vi "VI Tree.vi"   [LabVIEW 2010, in "Newport ESP301.lvlib"]
doc: "This is the instrument driver for the <INSTRUMENT NAME>. The VI Tree displays all the user-callable VIs of the instrument driver in an organized table.\n\nNOTE :\nEvery VIs need the VISA Ressource Name parameter for working."
uses:
  <userlib>/Newport ESP301/Newport ESP301.lvlib
panel:
  # "(c) 2009 <Newport>.  ALL RIGHTS RESERVED."
  # "SEE DIAGRAM\nFOR VI TREE."
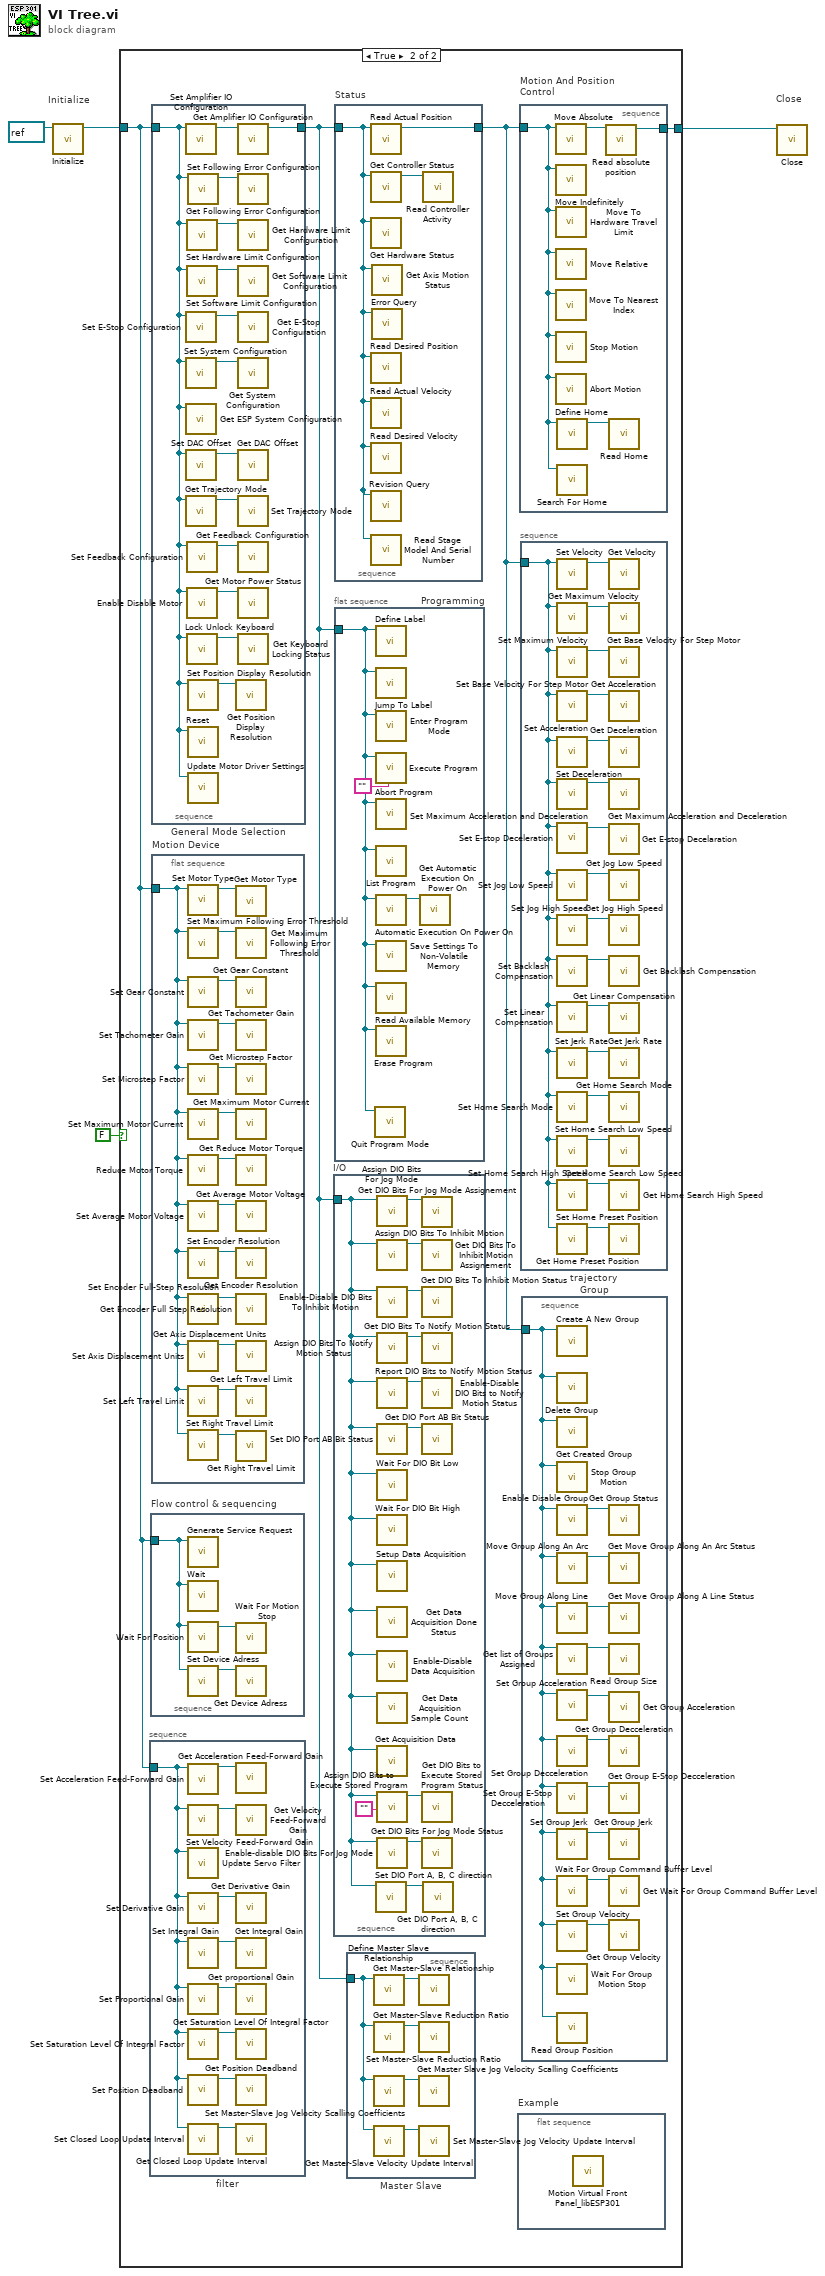
[diagram p0: block diagram]
diagram:
  # "Close"
  # "Initialize"
  n1 = call <userlib>:"Initialize.vi"("VISA resource name"=refnum<visa-resource-name> refnum) -> ("VISA resource name out"=w3:refnum<visa-resource-name>)  [unwired: 8 in, 1 out]
  n2 = case shown="True" FALSE {
    tunnel: w3 -> [w5 w8]
    tunnel: [w5 w6] -> w2
    frame False {
    }
    frame True {
      n3 = stacked-sequence "filter" {
        tunnel: w8 -> [w65]
        frame #0 {
          n4 = call <userlib>:"Set Acceleration Feed-Forward Gain.vi"("VISA resource name"=w65) -> ("VISA resource name out"=w66:refnum<visa-resource-name>)  [unwired: 5 in, 1 out]
          n5 = call <userlib>:"Set Velocity Feed-Forward Gain.vi"("VISA resource name"=w65) -> ("VISA resource name out"=w67:refnum<visa-resource-name>)  [unwired: 5 in, 1 out]
          n6 = call <userlib>:"Update Servo Filter.vi"("VISA resource name"=w65) -> ()  [unwired: 5 in, 2 out]
          n7 = call <userlib>:"Set Derivative Gain.vi"("VISA resource name"=w65) -> ("VISA resource name out"=w71:refnum<visa-resource-name>)  [unwired: 5 in, 1 out]
          n8 = call <userlib>:"Set Integral Gain.vi"("VISA resource name"=w65) -> ("VISA resource name out"=w72:refnum<visa-resource-name>)  [unwired: 5 in, 1 out]
          n9 = call <userlib>:"Set Proportional Gain.vi"("VISA resource name"=w65) -> ("VISA resource name out"=w70:refnum<visa-resource-name>)  [unwired: 5 in, 1 out]
          n10 = call <userlib>:"Set Saturation Level Of Integral Factor.vi"("VISA resource name"=w65) -> ("VISA resource name out"=w69:refnum<visa-resource-name>)  [unwired: 5 in, 1 out]
          n11 = call <userlib>:"Set Position Deadband.vi"("VISA resource name"=w65) -> ("VISA resource name out"=w68:refnum<visa-resource-name>)  [unwired: 5 in, 1 out]
          n12 = call <userlib>:"Set Closed Loop Update Interval.vi"("VISA resource name"=w65) -> ("VISA resource name out"=w64:refnum<visa-resource-name>)  [unwired: 5 in, 1 out]
          n13 = call <userlib>:"Get Acceleration Feed-Forward Gain.vi"("VISA resource name"=w66) -> ()  [unwired: 4 in, 3 out]
          n14 = call <userlib>:"Get Velocity Feed-Forward Gain.vi"("VISA resource name"=w67) -> ()  [unwired: 4 in, 3 out]
          n15 = call <userlib>:"Get Derivative Gain.vi"("VISA resource name"=w71) -> ()  [unwired: 4 in, 3 out]
          n16 = call <userlib>:"Get Integral Gain.vi"("VISA resource name"=w72) -> ()  [unwired: 4 in, 3 out]
          n17 = call <userlib>:"Get proportional Gain.vi"("VISA resource name"=w70) -> ()  [unwired: 4 in, 3 out]
          n18 = call <userlib>:"Get Saturation Level Of Integral Factor.vi"("VISA resource name"=w69) -> ()  [unwired: 4 in, 3 out]
          n19 = call <userlib>:"Get Position Deadband.vi"("VISA resource name"=w68) -> ()  [unwired: 4 in, 3 out]
          n20 = call <userlib>:"Get Closed Loop Update Interval.vi"("VISA resource name"=w64) -> ()  [unwired: 4 in, 3 out]
        }
      }
      n21 = stacked-sequence "Flow control & sequencing" {
        tunnel: w8 -> [w36]
        frame #0 {
          n22 = call <userlib>:"Generate Service Request.vi"("VISA resource name"=w36) -> ()  [unwired: 5 in, 2 out]
          n23 = call <userlib>:"Wait.vi"("VISA resource name"=w36) -> ()  [unwired: 5 in, 2 out]
          n24 = call <userlib>:"Wait For Position.vi"("VISA resource name"=w36) -> ("VISA resource name out"=w38:refnum<visa-resource-name>)  [unwired: 5 in, 1 out]
          n25 = call <userlib>:"Set Device Adress.vi"("VISA resource name"=w36) -> ("VISA resource name out"=w37:refnum<visa-resource-name>)  [unwired: 5 in, 1 out]
          n26 = call <userlib>:"Wait For Motion Stop.vi"("VISA resource name"=w38) -> ()  [unwired: 5 in, 2 out]
          n27 = call <userlib>:"Get Device Adress.vi"("VISA resource name"=w37) -> ()  [unwired: 4 in, 3 out]
        }
      }
      n28 = stacked-sequence "General Mode Selection" {
        tunnel: w8 -> [w23]
        tunnel: [w22] -> w7
        frame #0 {
          n29 = call <userlib>:"Set Amplifier IO Configuration.vi"("VISA resource name"=w23) -> ("VISA resource name out"=w31:refnum<visa-resource-name>)  [unwired: 5 in, 1 out]
          n30 = call <userlib>:"Set E-Stop Configuration.vi"("VISA resource name"=w23) -> ("VISA resource name out"=w32:refnum<visa-resource-name>)  [unwired: 5 in, 1 out]
          n31 = call <userlib>:"Set System Configuration.vi"("VISA resource name"=w23) -> ("VISA resource name out"=w28:refnum<visa-resource-name>)  [unwired: 5 in, 1 out]
          n32 = call <userlib>:"Get ESP System Configuration.vi"("VISA resource name"=w23) -> ()  [unwired: 4 in, 3 out]
          n33 = call <userlib>:"Set DAC Offset.vi"("VISA resource name"=w23) -> ("VISA resource name out"=w30:refnum<visa-resource-name>)  [unwired: 5 in, 1 out]
          n34 = call <userlib>:"Get Trajectory Mode.vi"("VISA resource name"=w23) -> ("VISA resource name out"=w29:refnum<visa-resource-name>)  [unwired: 4 in, 2 out]
          n35 = call <userlib>:"Set Hardware Limit Configuration.vi"("VISA resource name"=w23) -> ("VISA resource name out"=w35:refnum<visa-resource-name>)  [unwired: 5 in, 1 out]
          n36 = call <userlib>:"Set Software Limit Configuration.vi"("VISA resource name"=w23) -> ("VISA resource name out"=w33:refnum<visa-resource-name>)  [unwired: 5 in, 1 out]
          n37 = call <userlib>:"Set Feedback Configuration.vi"("VISA resource name"=w23) -> ("VISA resource name out"=w27:refnum<visa-resource-name>)  [unwired: 5 in, 1 out]
          n38 = call <userlib>:"Enable Disable Motor.vi"("VISA resource name"=w23) -> ("VISA resource name out"=w26:refnum<visa-resource-name>)  [unwired: 5 in, 1 out]
          n39 = call <userlib>:"Lock Unlock Keyboard.vi"("VISA resource name"=w23) -> ("VISA resource name out"=w25:refnum<visa-resource-name>)  [unwired: 5 in, 1 out]
          n40 = call <userlib>:"Set Following Error Configuration.vi"("VISA resource name"=w23) -> ("VISA resource name out"=w34:refnum<visa-resource-name>)  [unwired: 5 in, 1 out]
          n41 = call <userlib>:"Set Position Display Resolution.vi"("VISA resource name"=w23) -> ("VISA resource name out"=w24:refnum<visa-resource-name>)  [unwired: 5 in, 1 out]
          n42 = call <userlib>:"Reset.vi"("VISA resource name"=w23) -> ()  [unwired: 5 in, 2 out]
          n43 = call <userlib>:"Update Motor Driver Settings.vi"("VISA resource name"=w23) -> ()  [unwired: 5 in, 2 out]
          n44 = call <userlib>:"Get Position Display Resolution.vi"("VISA resource name"=w24) -> ()  [unwired: 4 in, 3 out]
          n45 = call <userlib>:"Get Amplifier IO Configuration.vi"("VISA resource name"=w31) -> ("VISA resource name out"=w22:refnum<visa-resource-name>)  [unwired: 4 in, 2 out]
          n46 = call <userlib>:"Get Following Error Configuration.vi"("VISA resource name"=w34) -> ()  [unwired: 4 in, 3 out]
          n47 = call <userlib>:"Get Hardware Limit Configuration.vi"("VISA resource name"=w35) -> ()  [unwired: 4 in, 3 out]
          n48 = call <userlib>:"Get Software Limit Configuration.vi"("VISA resource name"=w33) -> ()  [unwired: 4 in, 3 out]
          n49 = call <userlib>:"Get E-Stop Configuration.vi"("VISA resource name"=w32) -> ()  [unwired: 4 in, 3 out]
          n50 = call <userlib>:"Get System Configuration.vi"("VISA resource name"=w28) -> ()  [unwired: 4 in, 3 out]
          n51 = call <userlib>:"Get DAC Offset.vi"("VISA resource name"=w30) -> ()  [unwired: 4 in, 3 out]
          n52 = call <userlib>:"Set Trajectory Mode.vi"("VISA resource name"=w29) -> ()  [unwired: 6 in, 2 out]
          n53 = call <userlib>:"Get Feedback Configuration.vi"("VISA resource name"=w27) -> ()  [unwired: 4 in, 3 out]
          n54 = call <userlib>:"Get Motor Power Status.vi"("VISA resource name"=w26) -> ()  [unwired: 4 in, 3 out]
          n55 = call <userlib>:"Get Keyboard Locking Status.vi"("VISA resource name"=w25) -> ()  [unwired: 4 in, 3 out]
        }
      }
      n56 = flat-sequence "Motion Device" {
        tunnel: w8 -> [w91]
        frame #0 {
          n57 = call <userlib>:"Set Motor Type.vi"("VISA resource name"=w91) -> ("VISA resource name out"=w103:refnum<visa-resource-name>)  [unwired: 6 in, 1 out]
          n58 = call <userlib>:"Set Maximum Following Error Threshold.vi"("VISA resource name"=w91) -> ("VISA resource name out"=w102:refnum<visa-resource-name>)  [unwired: 5 in, 1 out]
          n59 = call <userlib>:"Set Gear Constant.vi"("VISA resource name"=w91) -> ("VISA resource name out"=w99:refnum<visa-resource-name>)  [unwired: 5 in, 1 out]
          n60 = call <userlib>:"Set Tachometer Gain.vi"("VISA resource name"=w91) -> ("VISA resource name out"=w101:refnum<visa-resource-name>)  [unwired: 5 in, 1 out]
          n61 = call <userlib>:"Set Microstep Factor.vi"("VISA resource name"=w91) -> ("VISA resource name out"=w100:refnum<visa-resource-name>)  [unwired: 5 in, 1 out]
          n62 = call <userlib>:"Set Maximum Motor Current.vi"("VISA resource name"=w91) -> ("VISA resource name out"=w90:refnum<visa-resource-name>)  [unwired: 5 in, 1 out]
          n63 = call <userlib>:"Reduce Motor Torque.vi"("VISA resource name"=w91) -> ("VISA resource name out"=w98:refnum<visa-resource-name>)  [unwired: 6 in, 1 out]
          n64 = call <userlib>:"Set Average Motor Voltage.vi"("VISA resource name"=w91) -> ("VISA resource name out"=w97:refnum<visa-resource-name>)  [unwired: 5 in, 1 out]
          n65 = call <userlib>:"Set Encoder Resolution.vi"("VISA resource name"=w91) -> ("VISA resource name out"=w96:refnum<visa-resource-name>)  [unwired: 5 in, 1 out]
          n66 = call <userlib>:"Set Encoder Full-Step Resolution.vi"("VISA resource name"=w91) -> ("VISA resource name out"=w95:refnum<visa-resource-name>)  [unwired: 5 in, 1 out]
          n67 = call <userlib>:"Set Axis Displacement Units.vi"("VISA resource name"=w91) -> ("VISA resource name out"=w92:refnum<visa-resource-name>)  [unwired: 6 in, 1 out]
          n68 = call <userlib>:"Set Left Travel Limit.vi"("VISA resource name"=w91) -> ("VISA resource name out"=w94:refnum<visa-resource-name>)  [unwired: 5 in, 1 out]
          n69 = call <userlib>:"Set Right Travel Limit.vi"("VISA resource name"=w91) -> ("VISA resource name out"=w93:refnum<visa-resource-name>)  [unwired: 5 in, 1 out]
          n70 = call <userlib>:"Get Motor Type.vi"("VISA resource name"=w103) -> ()  [unwired: 4 in, 3 out]
          n71 = call <userlib>:"Get Maximum Following Error Threshold.vi"("VISA resource name"=w102) -> ()  [unwired: 4 in, 3 out]
          n72 = call <userlib>:"Get Gear Constant.vi"("VISA resource name"=w99) -> ()  [unwired: 4 in, 3 out]
          n73 = call <userlib>:"Get Tachometer Gain.vi"("VISA resource name"=w101) -> ()  [unwired: 4 in, 3 out]
          n74 = call <userlib>:"Get Microstep Factor.vi"("VISA resource name"=w100) -> ()  [unwired: 4 in, 3 out]
          n75 = call <userlib>:"Get Maximum Motor Current.vi"("VISA resource name"=w90) -> ()  [unwired: 4 in, 3 out]
          n76 = call <userlib>:"Get Reduce Motor Torque.vi"("VISA resource name"=w98) -> ()  [unwired: 4 in, 3 out]
          n77 = call <userlib>:"Get Average Motor Voltage.vi"("VISA resource name"=w97) -> ()  [unwired: 4 in, 3 out]
          n78 = call <userlib>:"Get Encoder Resolution.vi"("VISA resource name"=w96) -> ()  [unwired: 4 in, 3 out]
          n79 = call <userlib>:"Get Encoder Full Step Resolution.vi"("VISA resource name"=w95) -> ()  [unwired: 4 in, 3 out]
          n80 = call <userlib>:"Get Axis Displacement Units.vi"("VISA resource name"=w92) -> ()  [unwired: 4 in, 3 out]
          n81 = call <userlib>:"Get Left Travel Limit.vi"("VISA resource name"=w94) -> ()  [unwired: 4 in, 3 out]
          n82 = call <userlib>:"Get Right Travel Limit.vi"("VISA resource name"=w93) -> ()  [unwired: 4 in, 3 out]
        }
      }
      n83 = stacked-sequence "I/O" {
        tunnel: w7 -> [w42]
        frame #0 {
          n84 = call <userlib>:"Set DIO Port A, B, C direction.vi"("VISA resource name"=w42) -> ("VISA resource name out"=w43:refnum<visa-resource-name>)  [unwired: 9 in, 1 out]
          n85 = call <userlib>:"Assign DIO Bits For Jog Mode.vi"("VISA resource name"=w42) -> ("VISA resource name out"=w52:refnum<visa-resource-name>)  [unwired: 6 in, 1 out]
          n86 = call <userlib>:"Assign DIO Bits To Inhibit Motion.vi"("VISA resource name"=w42) -> ("VISA resource name out"=w47:refnum<visa-resource-name>)  [unwired: 6 in, 1 out]
          n87 = call <userlib>:"Enable-Disable DIO Bits To Inhibit Motion.vi"("VISA resource name"=w42) -> ("VISA resource name out"=w48:refnum<visa-resource-name>)  [unwired: 5 in, 1 out]
          n88 = call <userlib>:"Assign DIO Bits To Notify Motion Status.vi"("VISA resource name"=w42) -> ("VISA resource name out"=w49:refnum<visa-resource-name>)  [unwired: 6 in, 1 out]
          n89 = call <userlib>:"Report DIO Bits to Notify Motion Status.vi"("VISA resource name"=w42) -> ("VISA resource name out"=w51:refnum<visa-resource-name>)  [unwired: 4 in, 2 out]
          n90 = call <userlib>:"Set DIO Port AB Bit Status.vi"("VISA resource name"=w42) -> ("VISA resource name out"=w50:refnum<visa-resource-name>)  [unwired: 5 in, 1 out]
          n91 = call <userlib>:"Wait For DIO Bit Low.vi"("VISA resource name"=w42) -> ()  [unwired: 5 in, 2 out]
          n92 = call <userlib>:"Wait For DIO Bit High.vi"("VISA resource name"=w42) -> ()  [unwired: 5 in, 2 out]
          n93 = call <userlib>:"Setup Data Acquisition.vi"("VISA resource name"=w42) -> ()  [unwired: 5 in, 2 out]
          n94 = call <userlib>:"Get Data Acquisition Done Status.vi"("VISA resource name"=w42) -> ()  [unwired: 4 in, 3 out]
          n95 = call <userlib>:"Enable-Disable Data Acquisition.vi"("VISA resource name"=w42) -> ()  [unwired: 5 in, 2 out]
          n96 = call <userlib>:"Get Data Acquisition Sample Count.vi"("VISA resource name"=w42) -> ()  [unwired: 4 in, 3 out]
          n97 = call <userlib>:"Get Acquisition Data.vi"("VISA resource name"=w42) -> ()  [unwired: 4 in, 3 out]
          n98 = call <userlib>:"Assign DIO Bits to Execute Stored Program.vi"("Program Name"="", "VISA resource name"=w42) -> ("VISA resource name out"=w46:refnum<visa-resource-name>)  [unwired: 4 in, 1 out]
          n99 = call <userlib>:"Enable-disable DIO Bits For Jog Mode.vi"("VISA resource name"=w42) -> ("VISA resource name out"=w44:refnum<visa-resource-name>)  [unwired: 5 in, 1 out]
          n100 = call <userlib>:"Get DIO Bits For Jog Mode Assignement.vi"("VISA resource name"=w52) -> ()  [unwired: 3 in, 4 out]
          n101 = call <userlib>:"Get DIO Bits To Inhibit Motion Assignement.vi"("VISA resource name"=w47) -> ()  [unwired: 3 in, 4 out]
          n102 = call <userlib>:"Get DIO Bits To Inhibit Motion Status.vi"("VISA resource name"=w48) -> ()  [unwired: 4 in, 3 out]
          n103 = call <userlib>:"Get DIO Bits To Notify Motion Status.vi"("VISA resource name"=w49) -> ()  [unwired: 3 in, 4 out]
          n104 = call <userlib>:"Enable-Disable DIO Bits to Notify Motion Status.vi"("VISA resource name"=w51) -> ()  [unwired: 5 in, 2 out]
          n105 = call <userlib>:"Get DIO Port AB Bit Status.vi"("VISA resource name"=w50) -> ()  [unwired: 4 in, 3 out]
          n106 = call <userlib>:"Get DIO Bits to Execute Stored Program Status.vi"("VISA resource name"=w46) -> ()  [unwired: 4 in, 3 out]
          n107 = call <userlib>:"Get DIO Bits For Jog Mode Status.vi"("VISA resource name"=w44) -> ()  [unwired: 4 in, 3 out]
          n108 = call <userlib>:"Get DIO Port A, B, C direction.vi"("VISA resource name"=w43) -> ()  [unwired: 8 in, 3 out]
        }
      }
      n109 = stacked-sequence "Status" {
        tunnel: w7 -> [w15]
        tunnel: [w14] -> w9
        frame #0 {
          n110 = call <userlib>:"Read Actual Position.vi"("VISA resource name"=w15) -> ("VISA resource name out"=w14:refnum<visa-resource-name>)  [unwired: 4 in, 2 out]
          n111 = call <userlib>:"Get Controller Status.vi"("VISA resource name"=w15) -> ("VISA resource name out"=w16:refnum<visa-resource-name>)  [unwired: 3 in, 3 out]
          n112 = call <userlib>:"Get Hardware Status.vi"("VISA resource name"=w15) -> ()  [unwired: 3 in, 4 out]
          n113 = call <userlib>:"Read Desired Position.vi"("VISA resource name"=w15) -> ()  [unwired: 4 in, 3 out]
          n114 = call <userlib>:"Read Actual Velocity.vi"("VISA resource name"=w15) -> ()  [unwired: 4 in, 3 out]
          n115 = call <userlib>:"Read Desired Velocity.vi"("VISA resource name"=w15) -> ()  [unwired: 4 in, 3 out]
          n116 = call <userlib>:"Revision Query.vi"("VISA resource name"=w15) -> ()  [unwired: 7 in, 4 out]
          n117 = call <userlib>:"Read Stage Model And Serial Number.vi"("VISA resource name"=w15) -> ()  [unwired: 3 in, 4 out]
          n118 = call <userlib>:"Get Axis Motion Status.vi"("VISA resource name"=w15) -> ()  [unwired: 4 in, 3 out]
          n119 = call <userlib>:"Error Query.vi"("VISA resource name"=w15) -> ()  [unwired: 3 in, 4 out]
          n120 = call <userlib>:"Read Controller Activity.vi"("VISA resource name"=w16) -> ()  [unwired: 4 in, 3 out]
        }
      }
      n121 = flat-sequence "Programming" {
        tunnel: w7 -> [w39]
        frame #0 {
          n122 = call <userlib>:"Quit Program Mode.vi"("VISA resource name"=w39) -> ()  [unwired: 5 in, 2 out]
          n123 = call <userlib>:"Define Label.vi"("VISA resource name"=w39) -> ()  [unwired: 5 in, 2 out]
          n124 = call <userlib>:"Jump To Label.vi"("VISA resource name"=w39) -> ()  [unwired: 5 in, 2 out]
          n125 = call <userlib>:"Enter Program Mode.vi"("VISA resource name"=w39) -> ()  [unwired: 5 in, 2 out]
          n126 = call <userlib>:"Execute Program.vi"("Program Name"="", "VISA resource name"=w39) -> ()  [unwired: 4 in, 2 out]
          n127 = call <userlib>:"Abort Program.vi"("VISA resource name"=w39) -> ()  [unwired: 5 in, 2 out]
          n128 = call <userlib>:"List Program.vi"("VISA resource name"=w39) -> ()  [unwired: 4 in, 3 out]
          n129 = call <userlib>:"Automatic Execution On Power On.vi"("VISA resource name"=w39) -> ("VISA resource name out"=w40:refnum<visa-resource-name>)  [unwired: 5 in, 1 out]
          n130 = call <userlib>:"Save Settings To Non-Volatile Memory.vi"("VISA resource name"=w39) -> ()  [unwired: 5 in, 2 out]
          n131 = call <userlib>:"Read Available Memory.vi"("VISA resource name"=w39) -> ()  [unwired: 5 in, 2 out]
          n132 = call <userlib>:"Erase Program.vi"("VISA resource name"=w39) -> ()  [unwired: 5 in, 2 out]
          n133 = call <userlib>:"Get Automatic Execution On Power On.vi"("VISA resource name"=w40) -> ()  [unwired: 3 in, 4 out]
        }
      }
      n134 = stacked-sequence "Master Slave" {
        tunnel: w7 -> [w17]
        frame #0 {
          n135 = call <userlib>:"Define Master Slave Relationship.vi"("VISA resource name"=w17) -> ("VISA resource name out"=w21:refnum<visa-resource-name>)  [unwired: 5 in, 1 out]
          n136 = call <userlib>:"Get Master-Slave Reduction Ratio.vi"("VISA resource name"=w17) -> ("VISA resource name out"=w20:refnum<visa-resource-name>)  [unwired: 4 in, 2 out]
          n137 = call <userlib>:"Set Master-Slave Jog Velocity Scalling Coefficients.vi"("VISA resource name"=w17) -> ("VISA resource name out"=w18:refnum<visa-resource-name>)  [unwired: 5 in, 1 out]
          n138 = call <userlib>:"Get Master-Slave Velocity Update Interval.vi"("VISA resource name"=w17) -> ("VISA resource name out"=w19:refnum<visa-resource-name>)  [unwired: 4 in, 2 out]
          n139 = call <userlib>:"Get Master-Slave Relationship.vi"("VISA resource name"=w21) -> ()  [unwired: 4 in, 3 out]
          n140 = call <userlib>:"Set Master-Slave Reduction Ratio.vi"("VISA resource name"=w20) -> ()  [unwired: 5 in, 2 out]
          n141 = call <userlib>:"Get Master Slave Jog Velocity Scalling Coefficients.vi"("VISA resource name"=w18) -> ()  [unwired: 3 in, 4 out]
          n142 = call <userlib>:"Set Master-Slave Jog Velocity Update Interval.vi"("VISA resource name"=w19) -> ()  [unwired: 5 in, 2 out]
        }
      }
      n143 = flat-sequence "Example" {
        frame #0 {
          n144 = call <userlib>:"Motion Virtual Front Panel_libESP301.vi"() -> ()  [unwired: 1 in]
        }
      }
      n145 = stacked-sequence "Motion And Position \nControl" {
        tunnel: w9 -> [w12]
        tunnel: [w10] -> w6
        frame #0 {
          n146 = call <userlib>:"Move Absolute.vi"("VISA resource name"=w12) -> ("VISA resource name out"=w13:refnum<visa-resource-name>)  [unwired: 5 in, 1 out]
          n147 = call <userlib>:"Move Indefinitely.vi"("VISA resource name"=w12) -> ()  [unwired: 5 in, 2 out]
          n148 = call <userlib>:"Move To Hardware Travel Limit.vi"("VISA resource name"=w12) -> ()  [unwired: 5 in, 2 out]
          n149 = call <userlib>:"Move Relative.vi"("VISA resource name"=w12) -> ()  [unwired: 5 in, 2 out]
          n150 = call <userlib>:"Move To Nearest Index.vi"("VISA resource name"=w12) -> ()  [unwired: 5 in, 2 out]
          n151 = call <userlib>:"Stop Motion.vi"("VISA resource name"=w12) -> ()  [unwired: 5 in, 2 out]
          n152 = call <userlib>:"Abort Motion.vi"("VISA resource name"=w12) -> ()  [unwired: 5 in, 2 out]
          n153 = call <userlib>:"Define Home.vi"("VISA resource name"=w12) -> ("VISA resource name out"=w11:refnum<visa-resource-name>)  [unwired: 5 in, 1 out]
          n154 = call <userlib>:"Search For Home.vi"("VISA resource name"=w12) -> ()  [unwired: 6 in, 2 out]
          n155 = call <userlib>:"Read absolute position.vi"("VISA resource name"=w13) -> ("VISA resource name out"=w10:refnum<visa-resource-name>)  [unwired: 4 in, 2 out]
          n156 = call <userlib>:"Read Home.vi"("VISA resource name"=w11) -> ()  [unwired: 4 in, 3 out]
        }
      }
      n157 = stacked-sequence "trajectory" {
        tunnel: w9 -> [w73]
        frame #0 {
          n158 = call <userlib>:"Set Velocity.vi"("VISA resource name"=w73) -> ("VISA resource name out"=w89:refnum<visa-resource-name>)  [unwired: 5 in, 1 out]
          n159 = call <userlib>:"Set Maximum Velocity.vi"("VISA resource name"=w73) -> ("VISA resource name out"=w88:refnum<visa-resource-name>)  [unwired: 5 in, 1 out]
          n160 = call <userlib>:"Set Base Velocity For Step Motor.vi"("VISA resource name"=w73) -> ("VISA resource name out"=w87:refnum<visa-resource-name>)  [unwired: 5 in, 1 out]
          n161 = call <userlib>:"Set Acceleration.vi"("VISA resource name"=w73) -> ("VISA resource name out"=w85:refnum<visa-resource-name>)  [unwired: 5 in, 1 out]
          n162 = call <userlib>:"Set Deceleration.vi"("VISA resource name"=w73) -> ("VISA resource name out"=w86:refnum<visa-resource-name>)  [unwired: 5 in, 1 out]
          n163 = call <userlib>:"Set Maximum Acceleration and Deceleration.vi"("VISA resource name"=w73) -> ("VISA resource name out"=w84:refnum<visa-resource-name>)  [unwired: 5 in, 1 out]
          n164 = call <userlib>:"Set E-stop Deceleration.vi"("VISA resource name"=w73) -> ("VISA resource name out"=w83:refnum<visa-resource-name>)  [unwired: 5 in, 1 out]
          n165 = call <userlib>:"Set Jog Low Speed.vi"("VISA resource name"=w73) -> ("VISA resource name out"=w81:refnum<visa-resource-name>)  [unwired: 5 in, 1 out]
          n166 = call <userlib>:"Set Jog High Speed.vi"("VISA resource name"=w73) -> ("VISA resource name out"=w80:refnum<visa-resource-name>)  [unwired: 5 in, 1 out]
          n167 = call <userlib>:"Set Backlash Compensation.vi"("VISA resource name"=w73) -> ("VISA resource name out"=w82:refnum<visa-resource-name>)  [unwired: 5 in, 1 out]
          n168 = call <userlib>:"Set Linear Compensation.vi"("VISA resource name"=w73) -> ("VISA resource name out"=w78:refnum<visa-resource-name>)  [unwired: 5 in, 1 out]
          n169 = call <userlib>:"Set Jerk Rate.vi"("VISA resource name"=w73) -> ("VISA resource name out"=w79:refnum<visa-resource-name>)  [unwired: 5 in, 1 out]
          n170 = call <userlib>:"Set Home Search Mode.vi"("VISA resource name"=w73) -> ("VISA resource name out"=w74:refnum<visa-resource-name>)  [unwired: 6 in, 1 out]
          n171 = call <userlib>:"Set Home Search Low Speed.vi"("VISA resource name"=w73) -> ("VISA resource name out"=w75:refnum<visa-resource-name>)  [unwired: 5 in, 1 out]
          n172 = call <userlib>:"Set Home Search High Speed.vi"("VISA resource name"=w73) -> ("VISA resource name out"=w76:refnum<visa-resource-name>)  [unwired: 5 in, 1 out]
          n173 = call <userlib>:"Set Home Preset Position.vi"("VISA resource name"=w73) -> ("VISA resource name out"=w77:refnum<visa-resource-name>)  [unwired: 5 in, 1 out]
          n174 = call <userlib>:"Get Velocity.vi"("VISA resource name"=w89) -> ()  [unwired: 4 in, 3 out]
          n175 = call <userlib>:"Get Maximum Velocity.vi"("VISA resource name"=w88) -> ()  [unwired: 4 in, 3 out]
          n176 = call <userlib>:"Get Base Velocity For Step Motor.vi"("VISA resource name"=w87) -> ()  [unwired: 4 in, 3 out]
          n177 = call <userlib>:"Get Acceleration.vi"("VISA resource name"=w85) -> ()  [unwired: 4 in, 3 out]
          n178 = call <userlib>:"Get Deceleration.vi"("VISA resource name"=w86) -> ()  [unwired: 4 in, 3 out]
          n179 = call <userlib>:"Get Maximum Acceleration and Deceleration.vi"("VISA resource name"=w84) -> ()  [unwired: 4 in, 3 out]
          n180 = call <userlib>:"Get E-stop Decelaration.vi"("VISA resource name"=w83) -> ()  [unwired: 4 in, 3 out]
          n181 = call <userlib>:"Get Jog Low Speed.vi"("VISA resource name"=w81) -> ()  [unwired: 4 in, 3 out]
          n182 = call <userlib>:"Get Jog High Speed.vi"("VISA resource name"=w80) -> ()  [unwired: 4 in, 3 out]
          n183 = call <userlib>:"Get Backlash Compensation.vi"("VISA resource name"=w82) -> ()  [unwired: 4 in, 3 out]
          n184 = call <userlib>:"Get Linear Compensation.vi"("VISA resource name"=w78) -> ()  [unwired: 4 in, 3 out]
          n185 = call <userlib>:"Get Jerk Rate.vi"("VISA resource name"=w79) -> ()  [unwired: 4 in, 3 out]
          n186 = call <userlib>:"Get Home Search Mode.vi"("VISA resource name"=w74) -> ()  [unwired: 4 in, 3 out]
          n187 = call <userlib>:"Get Home Search Low Speed.vi"("VISA resource name"=w75) -> ()  [unwired: 4 in, 3 out]
          n188 = call <userlib>:"Get Home Search High Speed.vi"("VISA resource name"=w76) -> ()  [unwired: 4 in, 3 out]
          n189 = call <userlib>:"Get Home Preset Position.vi"("VISA resource name"=w77) -> ()  [unwired: 4 in, 3 out]
        }
      }
      n190 = stacked-sequence "Group" {
        tunnel: w9 -> [w53]
        frame #0 {
          n191 = call <userlib>:"Create A New Group.vi"("VISA resource name"=w53) -> ()  [unwired: 5 in, 2 out]
          n192 = call <userlib>:"Delete Group.vi"("VISA resource name"=w53) -> ()  [unwired: 5 in, 2 out]
          n193 = call <userlib>:"Get Created Group.vi"("VISA resource name"=w53) -> ()  [unwired: 4 in, 3 out]
          n194 = call <userlib>:"Stop Group Motion.vi"("VISA resource name"=w53) -> ()  [unwired: 5 in, 2 out]
          n195 = call <userlib>:"Enable Disable Group.vi"("VISA resource name"=w53) -> ("VISA resource name out"=w56:refnum<visa-resource-name>)  [unwired: 5 in, 1 out]
          n196 = call <userlib>:"Move Group Along An Arc.vi"("VISA resource name"=w53) -> ("VISA resource name out"=w54:refnum<visa-resource-name>)  [unwired: 5 in, 1 out]
          n197 = call <userlib>:"Move Group Along Line.vi"("VISA resource name"=w53) -> ("VISA resource name out"=w55:refnum<visa-resource-name>)  [unwired: 5 in, 1 out]
          n198 = call <userlib>:"Get list of Groups Assigned.vi"("VISA resource name"=w53) -> ("VISA resource name out"=w63:refnum<visa-resource-name>)  [unwired: 4 in, 2 out]
          n199 = call <userlib>:"Set Group Acceleration.vi"("VISA resource name"=w53) -> ("VISA resource name out"=w62:refnum<visa-resource-name>)  [unwired: 5 in, 1 out]
          n200 = call <userlib>:"Set Group Decceleration.vi"("VISA resource name"=w53) -> ("VISA resource name out"=w61:refnum<visa-resource-name>)  [unwired: 5 in, 1 out]
          n201 = call <userlib>:"Set Group E-Stop Decceleration.vi"("VISA resource name"=w53) -> ("VISA resource name out"=w60:refnum<visa-resource-name>)  [unwired: 5 in, 1 out]
          n202 = call <userlib>:"Set Group Jerk.vi"("VISA resource name"=w53) -> ("VISA resource name out"=w59:refnum<visa-resource-name>)  [unwired: 5 in, 1 out]
          n203 = call <userlib>:"Wait For Group Command Buffer Level.vi"("VISA resource name"=w53) -> ("VISA resource name out"=w58:refnum<visa-resource-name>)  [unwired: 5 in, 1 out]
          n204 = call <userlib>:"Set Group Velocity.vi"("VISA resource name"=w53) -> ("VISA resource name out"=w57:refnum<visa-resource-name>)  [unwired: 5 in, 1 out]
          n205 = call <userlib>:"Wait For Group Motion Stop.vi"("VISA resource name"=w53) -> ()  [unwired: 5 in, 2 out]
          n206 = call <userlib>:"Read Group Position.vi"("VISA resource name"=w53) -> ()  [unwired: 4 in, 3 out]
          n207 = call <userlib>:"Get Group Status.vi"("VISA resource name"=w56) -> ()  [unwired: 4 in, 3 out]
          n208 = call <userlib>:"Get Move Group Along An Arc Status.vi"("VISA resource name"=w54) -> ()  [unwired: 4 in, 3 out]
          n209 = call <userlib>:"Get Move Group Along A Line Status.vi"("VISA resource name"=w55) -> ()  [unwired: 4 in, 3 out]
          n210 = call <userlib>:"Read Group Size.vi"("VISA resource name"=w63) -> ()  [unwired: 4 in, 3 out]
          n211 = call <userlib>:"Get Group Acceleration.vi"("VISA resource name"=w62) -> ()  [unwired: 4 in, 3 out]
          n212 = call <userlib>:"Get Group Decceleration.vi"("VISA resource name"=w61) -> ()  [unwired: 4 in, 3 out]
          n213 = call <userlib>:"Get Group E-Stop Decceleration.vi"("VISA resource name"=w60) -> ()  [unwired: 4 in, 3 out]
          n214 = call <userlib>:"Get Group Jerk.vi"("VISA resource name"=w59) -> ()  [unwired: 4 in, 3 out]
          n215 = call <userlib>:"Get Wait For Group Command Buffer Level.vi"("VISA resource name"=w58) -> ()  [unwired: 4 in, 3 out]
          n216 = call <userlib>:"Get Group Velocity.vi"("VISA resource name"=w57) -> ()  [unwired: 4 in, 3 out]
        }
      }
    }
  }
  n217 = call <userlib>:"Close.vi"("VISA resource name"=w2) -> ()  [unwired: 10 in, 1 out]
